vi "Send SetAmplitudeRange.vi"(6 "reference level offset":dbl, 7 "Message Priority (Normal)":T1=enum."Normal", 8 "error in (no error)":errorcluster, 9 "Attenuation":dbl format="%#_13g", 10 "Ref Level":dbl format="%#_13g", 11 "Message Enqueuer":refnum<class "Message Enqueuer.lvclass">) -> (0 "error out":errorcluster, 3 "Message Enqueuer out":refnum<class "Message Enqueuer.lvclass">)   [LabVIEW 2023, in "SpectrumAnalyzerInterface.lvlib" / "SetAmplitudeRange Msg.lvclass"]
doc: "This VI sends the message to an actor."
uses:
  SetAmplitudeRange Msg.lvclass
  SetAmplitudeRange Msg.lvclass/SetAmplitudeRange Msg.ctl
  <vilib>/ActorFramework/Message Enqueuer/Message Enqueuer.lvclass
  C:/Program Files/National Instruments/LabVIEW 2023/vi.lib/ActorFramework/Message/Message.lvclass
  C:/Users/DELL/Desktop/SpectrumAnalyzer Messages/SetAmplitudeRange Msg/SetAmplitudeRange Msg.lvclass
  <vilib>/ActorFramework/Message Enqueuer/Message Priority.ctl
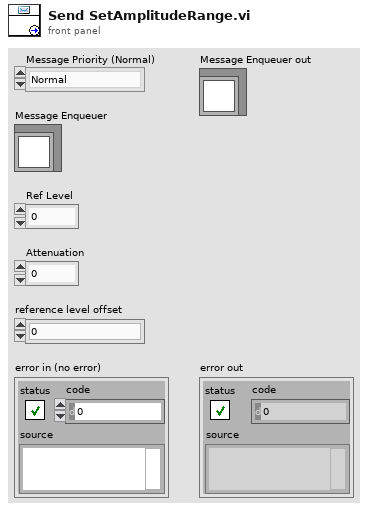
[diagram p1: front panel]
types:
  T1 = typedef "Actor Framework.lvlib/Message Enqueuer.lvclass/Message Priority.ctl" = enum16{"Low", "Normal", "High"}
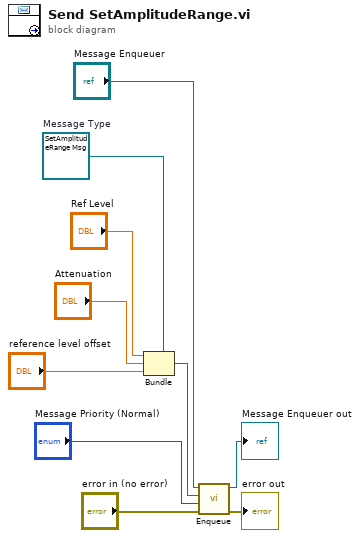
[diagram p0: block diagram]
diagram:
  w4 = refnum<class "SetAmplitudeRange Msg.lvclass"> refnum  # Message Type
  n1 = Bundle(cluster=w4, "Ref Level", "Attenuation", "reference level offset") -> (w5:refnum<class "SetAmplitudeRange Msg.lvclass">)
  n2 = call <vilib>:"Enqueue.vi"("error in (no error)"="error in (no error)", "Message Priority (Normal)"="Message Priority (Normal)", "Message"=w5, "Message Enqueuer in"="Message Enqueuer") -> ("error out"=→"error out":errorcluster, "Message Enqueuer in"=→"Message Enqueuer out":refnum<class "Message Enqueuer.lvclass">)  [unwired: 6 in]
